vi "Get Measurement Helper Library.vi"(8 "error in (no error)":errorcluster, 11 "Project in":refnum<vi>) -> (0 "error out":errorcluster, 2 "Found":bool, 3 "Library Item":refnum<vi>)   [LabVIEW 2020, in "MeasurementService Editor.lvlib"]
uses:
  MeasurementService Editor.lvlib
  <vilib>/Utility/Data Type/Type Definitions/Data Type.ctl
  <vilib>/Utility/Data Type/NI_Data Type.lvlib
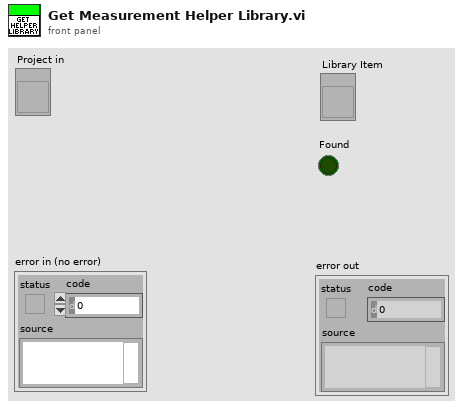
[diagram p1: front panel]
types:
  T1 = typedef "NI_Data Type.lvlib/Data Type.ctl" = enum8{"Invalid Type", "Void", "I8", "I16", "I32", "I64", "U8", "U16", "U32", "U64", "Single Float", "Double Float", "Extended Float", "Single Complex", "Double Complex", "Extended Complex", "Enum U8", "Enum U16", "Enum U32", "Enum U64", "Single Float With Unit", "Double Float With Unit", "Extended Float With Unit", "Single Complex with Unit", "Double Complex with Unit", "Extended Complex with Unit", "Boolean", "String", "Path", "Picture", "Tag", "Array", "Cluster", "Variant", "LV Variant", "Waveform", "Timestamp", "Digital Waveform", "Digital Data", "ExpressData", "Refnum", "External Data", "VI", "Poly VI", "LabVIEW Class Instance", "Fixed Point", "Set Collection", "Map Collection"}
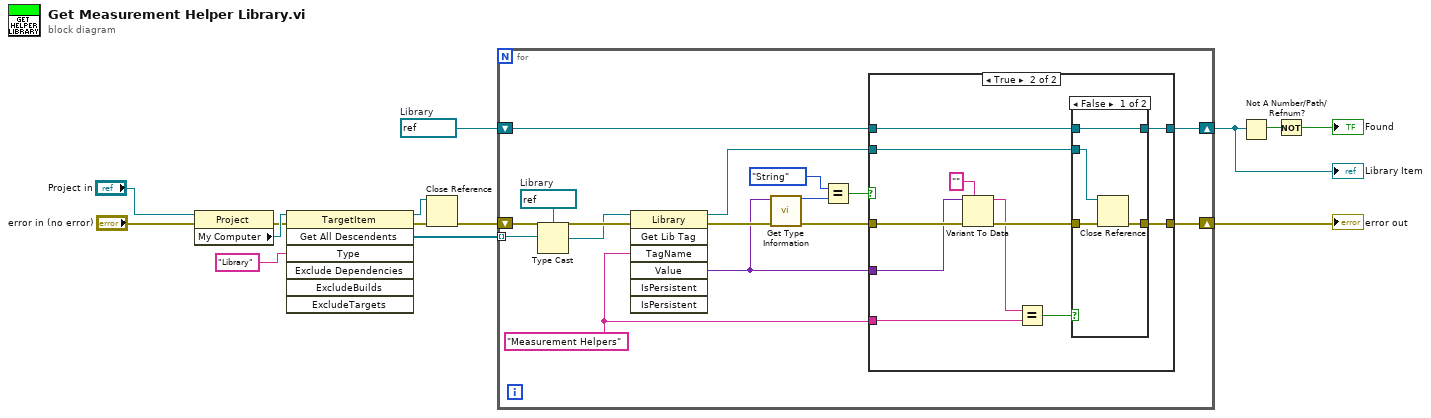
[diagram p0: block diagram]
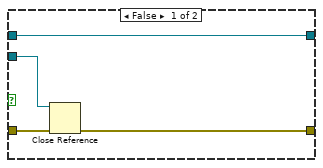
[diagram p2: hidden frame]
diagram:
  w8 = refnum<vi> refnum  # Library
  n1 = property class="Project"(reference="Project in", error in="error in (no error)") -> (error out=w13:errorcluster, "My Computer"=w14:refnum<vi>)  [unwired: 1 out]
  n2 = invoke class="TargetItem" method="Get All Descendents"(reference=w14, error in=w13, "Type"="Library") -> (reference out=w10:refnum<vi>, error out=w11:errorcluster, "All Descendents"=w12:refnum<vi>[])  [unwired: 4 in, 4 out]
  n3 = Close Reference(reference=w10, error in (no error)=w11) -> (error out=w9:errorcluster)
  n4 = for {
    tunnel: w12 -> [w22] mode=indexing
    shift-right: [w28] -> w2
    shift-left: w9 -> [w29]
    shift-right: [w27] -> w1
    shift-left: w8 -> [w26]
    w20 = refnum<vi> refnum  # Library
    w24 = "Measurement Helpers" ("Tag Name")
    n5 = Type Cast(type=w20, x=w22) -> (*(type *) &x=w21:refnum<vi>)
    n6 = invoke class="Library" method="Get Lib Tag"(reference=w21, error in=w29, "TagName"=w24) -> (reference out=w23:refnum<vi>, error out=w25:errorcluster, "Value"=w18:variant)  [unwired: 4 in, 4 out]
    n7 = call <vilib>:"Get Type Information.vi"("error in (no error)"=w25, "variant"=w18) -> ("error out"=w19:errorcluster, "type"=w17:T1)  [unwired: 5 in, 3 out]
    n8 = Equal?(x=Data_Type."String" ("type"), y=w17) -> (x = y?=w15:bool)
    n9 = case shown="True" w15 {
      tunnel: [w31 w44] -> w28
      tunnel: [w32 w43] -> w27
      tunnel: w26 -> [w32 w42]
      tunnel: w19 -> [w33 w41]
      tunnel: w24 -> [_ w40]
      tunnel: w18 -> [_ w37]
      tunnel: w23 -> [w30 w34]
      frame False {
        n10 = Close Reference(reference=w30, error in (no error)=w33) -> (error out=w31:errorcluster)
      }
      frame True {
        n11 = Variant To Data(error in=w41, type="", Variant=w37) -> (data=w35:string, error out=w38:errorcluster)
        n12 = Equal?(x=w35, y=w40) -> (x = y?=w39:bool)
        n13 = case shown="False" w39 {
          tunnel: w38 -> [w48 w50]
          tunnel: [w47 w50] -> w44
          tunnel: [w46 w49] -> w43
          tunnel: w42 -> [w46 _]
          tunnel: w34 -> [w45 w49]
          frame False {
            n14 = Close Reference(reference=w45, error in (no error)=w48) -> (error out=w47:errorcluster)
          }
          frame True {
          }
        }
      }
    }
  }
  "error out" <- w2
  "Library Item" <- w1
  n15 = Not A Number/Path/Refnum?(number/path/refnum=w1) -> (NaN/Path/Refnum?=w4:bool)
  n16 = Not(x=w4) -> (.not. x?=→"Found":bool)
